vi "KGN Get Pump Mode general.vi"(8 "Fehler (Eingang, kein Fehler)":errorcluster, 9 "Info Cluster":T4, 10 "VISA-Ressourcenname":refnum<visa-resource-name>, 11 "device (Eingang)":u32) -> (0 "Fehler (Ausgang)":errorcluster, 1 "Info Cluster out":T4, 2 "VISA-Ressourcenname out":refnum<visa-resource-name>, 3 "dup device (Ausgang)":u32, 4 "PumpModeGeneral-Cluster":T3 {"dry mode" items=["wet", "dry"]; "control mode" items=["static", "pid"]}, 6 "Kommandos gesendet":string)   [LabVIEW 2020, in "Linearisierung v2.lvlib" / "Gasteiler.lvlib" / "HovaCAL_Interface.lvlib" / "KGN.lvlib" / "KGN GUI Get.lvlib"]
uses:
  KGN GUI Get.lvlib
  Controls/Info Cluster.ctl
  Controls/Pump Dry Mode.ctl
  Controls/Pump Control Mode.ctl
  get/get.lvlib
  Controls/Controls.lvlib
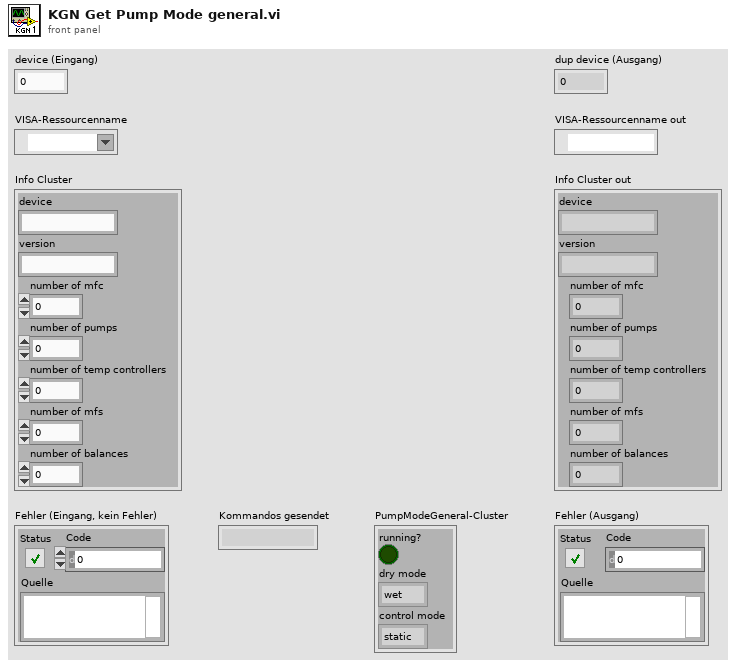
[diagram p1: front panel]
types:
  T1 = typedef "Linearisierung v2.lvlib/Gasteiler.lvlib/HovaCAL_Interface.lvlib/Controls.lvlib/Pump Dry Mode.ctl" = i32
  T2 = typedef "Linearisierung v2.lvlib/Gasteiler.lvlib/HovaCAL_Interface.lvlib/Controls.lvlib/Pump Control Mode.ctl" = u32
  T3 = cluster{"running?":bool, "dry mode":T1, "control mode":T2}
  T4 = typedef "Linearisierung v2.lvlib/Gasteiler.lvlib/HovaCAL_Interface.lvlib/Controls.lvlib/Info Cluster.ctl" = cluster{"device":string, "version":string, "number of mfc":i32, "number of pumps":i32, "number of temp controllers":i32, "number of mfs":i32, "number of balances":i32}
  T5 = cluster{"run":bool, "drywet":dbl, "control mode":dbl}
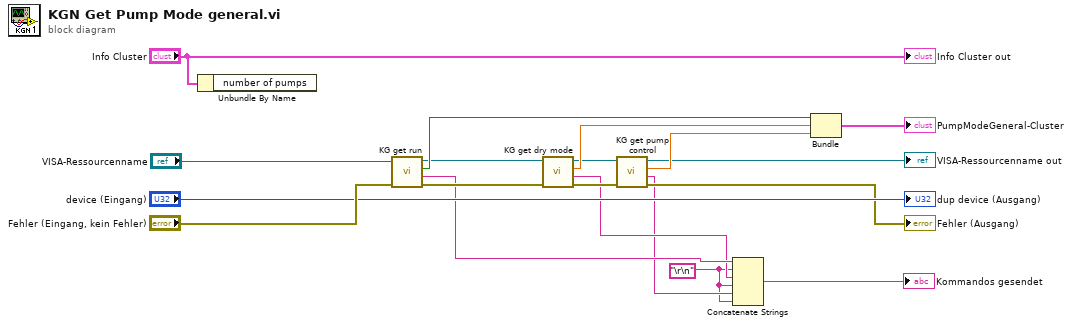
[diagram p0: block diagram]
diagram:
  w2 = "\r\n"
  n1 = Unbundle By Name("Info Cluster") -> ()  [unwired: 1 out]
  n2 = call "KG get run.vi"("Fehler (Eingang, kein Fehler)"="Fehler (Eingang, kein Fehler)", "VISA-Ressourcenname"="VISA-Ressourcenname") -> ("Fehler (Ausgang)"=w12:errorcluster, "Kommando gesendet"=w5:string, "run"=w16:bool, "VISA-Ressourcenname (Ausgang)"=w11:refnum<visa-resource-name>)  [unwired: 6 in]
  n3 = call "KG get dry mode.vi"("Fehler (Eingang, kein Fehler)"=w12, "VISA-Ressourcenname"=w11) -> ("Fehler (Ausgang)"=w7:errorcluster, "Kommando gesendet"=w4:string, "drywet"=w15:dbl, "VISA-Ressourcenname (Ausgang)"=w10:refnum<visa-resource-name>)  [unwired: 6 in]
  n4 = call "KG get pump control.vi"("Fehler (Eingang, kein Fehler)"=w7, "VISA-Ressourcenname"=w10) -> ("Fehler (Ausgang)"=→"Fehler (Ausgang)":errorcluster, "Kommando gesendet"=w3:string, "control mode"=w9:dbl, "VISA-Ressourcenname (Ausgang)"=→"VISA-Ressourcenname out":refnum<visa-resource-name>)  [unwired: 6 in]
  n5 = Concatenate Strings(w5, w2, w4, w2, w3, w2) -> (→"Kommandos gesendet":string)
  n6 = Bundle("run"=w16, "drywet"=w15, "control mode"=w9) -> (→"PumpModeGeneral-Cluster":T5)  [unwired: 1 in]
  "dup device (Ausgang)" <- "device (Eingang)"
  "Info Cluster out" <- "Info Cluster"
